vi "ZCAN_FilterSheet.vi"(0 "error in (no error)":errorcluster caption="错误输入（无错误）", 2 "can_index_handle":u32, 5 "can_index":u32, 7 "filter_mode":u32, 9 "filter_start":string, 11 "filter_end":string) -> (14 "error out":errorcluster caption="错误输出", 16 "can_index_handle（out）":u32, 19 "can_index (out)":u32)   [LabVIEW 2020, in "zlgcan.lvlib"]
uses:
  zlgcan.lvlib
  bin/zlgcan_wrap.dll
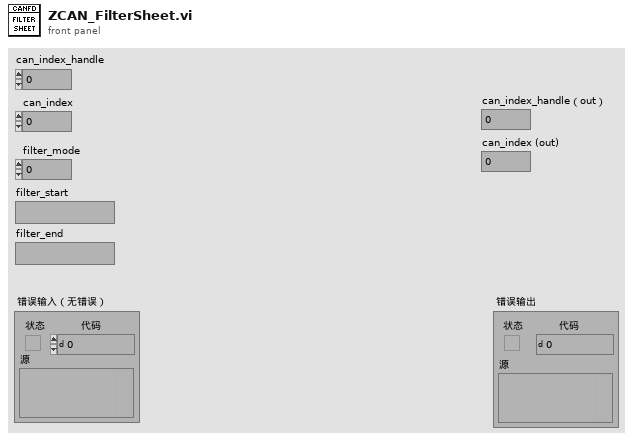
[diagram p1: front panel]
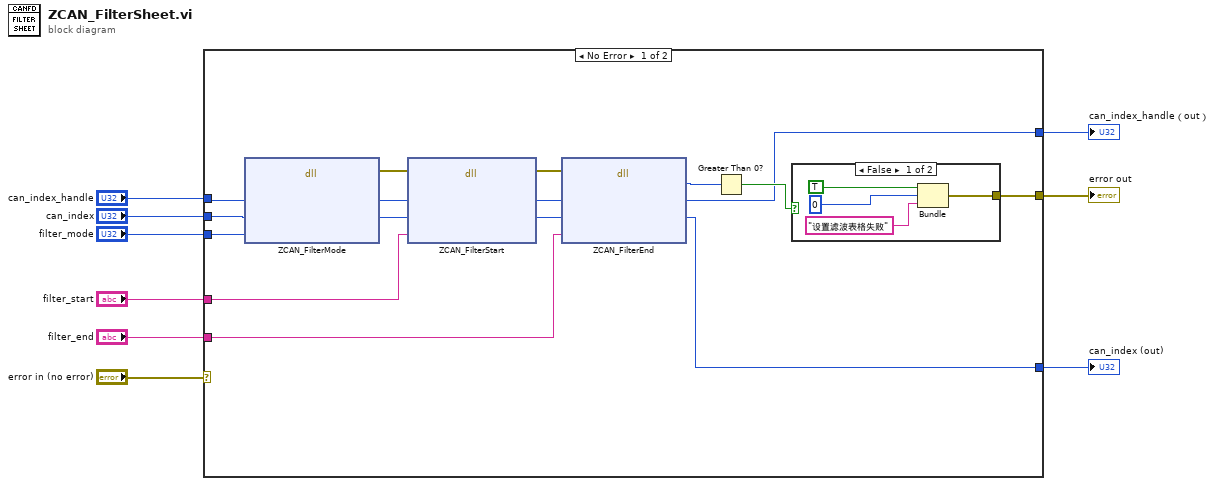
[diagram p0: block diagram]
diagram:
  n1 = case shown="No Error" "error in (no error)" {
    selector: "error in (no error)" -> [_ w30]
    tunnel: [w15 w30] -> w8
    tunnel: "can_index_handle" -> [w19 _]
    tunnel: "can_index" -> [w18 _]
    tunnel: "filter_mode" -> [w14 _]
    tunnel: "filter_start" -> [w13 _]
    tunnel: "filter_end" -> [w12 _]
    tunnel: [w11 _] -> w2
    tunnel: [w10 _] -> w1
    frame No Error {
      n2 = dll-call lib="E:/Jabil tools/JabilTestLib/LV/ZLG_CANFD/bin/zlgcan_wrap.dll" fn="ZCAN_FilterMode"("device_handle"=w19, "can_index"=w18, "mode"=w14) -> (error out=w20:errorcluster, "device_handle"=w21:u32, "can_index"=w22:u32)  [unwired: 5 in, 1 out]
      n3 = dll-call lib="E:/Jabil tools/JabilTestLib/LV/ZLG_CANFD/bin/zlgcan_wrap.dll" fn="ZCAN_FilterStart"(error in=w20, "device_handle"=w21, "can_index"=w22, "start"=w13) -> (error out=w25:errorcluster, "device_handle"=w23:u32, "can_index"=w24:u32)  [unwired: 4 in, 1 out]
      n4 = dll-call lib="E:/Jabil tools/JabilTestLib/LV/ZLG_CANFD/bin/zlgcan_wrap.dll" fn="ZCAN_FilterEnd"(error in=w25, "device_handle"=w23, "can_index"=w24, "end"=w12) -> ("return"=w17:u32, "device_handle"=w11:u32, "can_index"=w10:u32)  [unwired: 3 in, 2 out]
      n5 = Greater Than 0?(x=w17) -> (x > 0?=w16:bool)
      n6 = case shown="False" w16 {
        tunnel: [w26 _] -> w15
        frame False {
          n7 = Bundle("status"=TRUE, "code"=0, "消息"="设置滤波表格失败") -> (w26:cluster{"status":bool, "code":i32, "消息":string})  [unwired: 1 in]
        }
        frame True {
        }
      }
    }
    frame Error {
    }
  }
  "error out" <- w8
  "can_index_handle（out）" <- w2
  "can_index (out)" <- w1
